vi "Get Auth.vi"(11 "Async Authorization in":refnum<class "Async Authorization.lvclass">) -> (2 "Authorization":refnum<class "Authorization.lvclass">)   [LabVIEW 2020, in "OAuth2.lvlib" / "Async Authorization.lvclass"]
uses:
  Async Authorization.lvclass
  Authorization/Authorization.lvclass
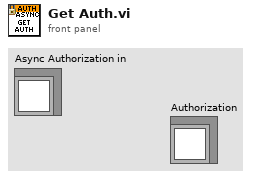
[diagram p1: front panel]
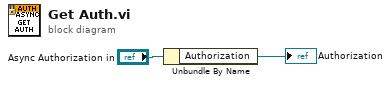
[diagram p0: block diagram]
diagram:
  n1 = Unbundle By Name("Async Authorization in") -> ("Authorization"=→"Authorization":refnum<class "Authorization.lvclass">)
